vi "Get Request Type.vi"(8 "error in (no error)":errorcluster, 11 "GetInputMute in":refnum<class "GetInputMute.lvclass">) -> (0 "error out":errorcluster, 2 "Request Type":string, 3 "GetInputMute out":refnum<class "GetInputMute.lvclass">)   [LabVIEW 2022 SP3, in "obs-websocket-lv.lvlib" / "GetInputMute.lvclass"]
uses:
  GetInputMute.lvclass
  GetInputMute.lvclass/GetInputMute.ctl
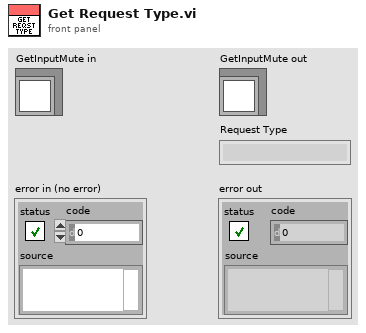
[diagram p1: front panel]
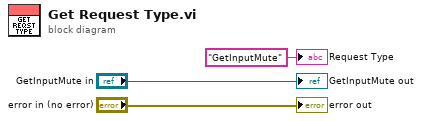
[diagram p0: block diagram]
diagram:
  "error out" <- "error in (no error)"
  "GetInputMute out" <- "GetInputMute in"
  "Request Type" <- "GetInputMute" ("Request Type")
